vi "ReadTriggerChannelCountNode.vi"(8 "Error In":errorcluster, 11 "Trigger Node In":refnum<k20>) -> (0 "Error Out":errorcluster, 1 "Infinite?":bool, 2 "Count":u32, 3 "Trigger Node Out":refnum<k20>, 5 "Auto?":bool)   [LabVIEW 2012]
uses:
  <vilib>/xml/NI_XML.lvlib
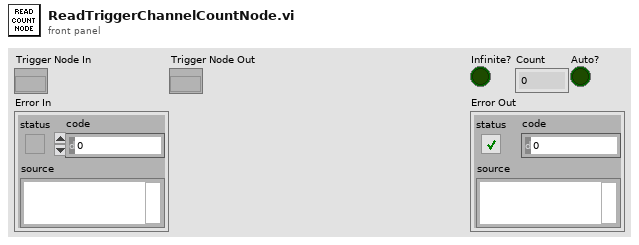
[diagram p1: front panel]
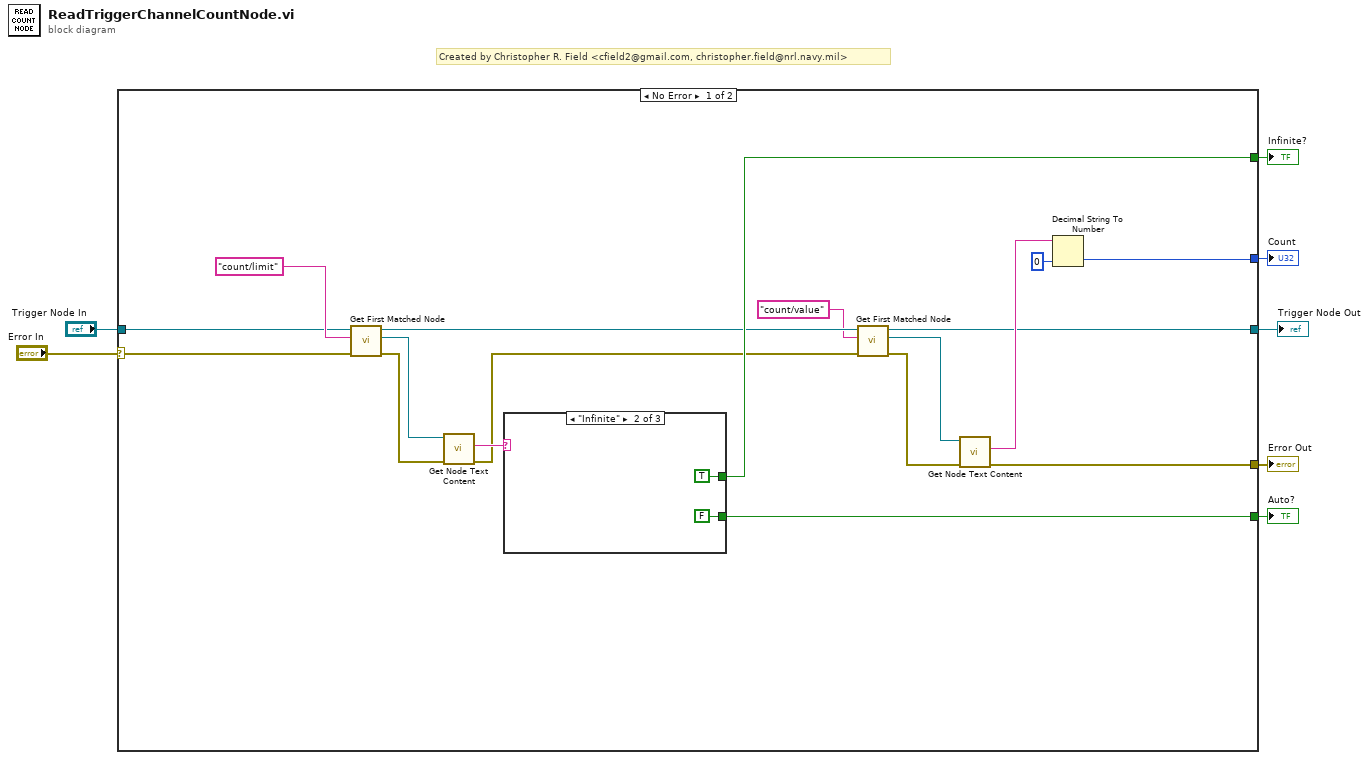
[diagram p0: block diagram]
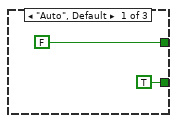
[diagram p2: hidden frame]
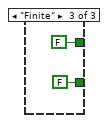
[diagram p3: hidden frame]
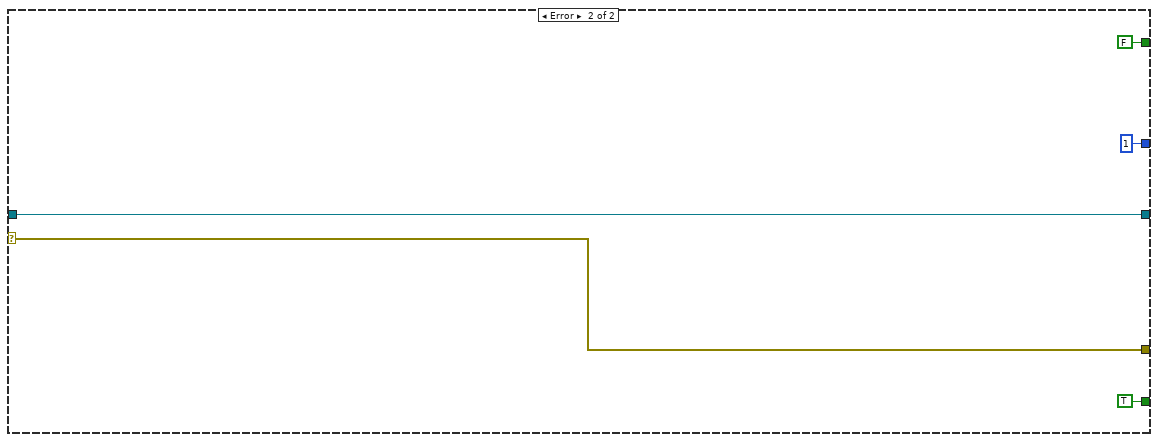
[diagram p4: hidden frame]
diagram:
  # "Created by Christopher R. Field <cfield2@gmail.com, christopher.field@nrl.navy.mil>"
  n1 = case shown="No Error" "Error In" {
    selector: "Error In" -> [w11 w36]
    tunnel: "Trigger Node In" -> [w12 w33]
    tunnel: [w21 FALSE] -> w5
    tunnel: [w13 u32 1] -> w4
    tunnel: [w10 w33] -> w3
    tunnel: [w9 w36] -> w2
    tunnel: [w8 TRUE] -> w1
    frame No Error {
      n2 = call <vilib>:"Get First Matched Node.vi"("error in (no error)"=w11, "XPath expression"="count/limit", "node in"=w12) -> ("error out"=w23:errorcluster, "node result"=w24:refnum<k20>, "node out"=w20:refnum<k20>)  [unwired: 6 in]
      n3 = call <vilib>:"Get Node Text Content.vi"("error in (no error)"=w23, "node in"=w24) -> ("error out"=w18:errorcluster, "node text"=w22:string)  [unwired: 7 in, 1 out]
      n4 = case shown="\"Infinite\"" w22 {
        tunnel: [FALSE TRUE FALSE] -> w21
        tunnel: [TRUE FALSE FALSE] -> w8
        frame "Auto", Default {
        }
        frame "Infinite" {
        }
        frame "Finite" {
        }
      }
      n5 = call <vilib>:"Get First Matched Node.vi"("error in (no error)"=w18, "XPath expression"="count/value", "node in"=w20) -> ("error out"=w16:errorcluster, "node result"=w17:refnum<k20>, "node out"=w10:refnum<k20>)  [unwired: 6 in]
      n6 = call <vilib>:"Get Node Text Content.vi"("error in (no error)"=w16, "node in"=w17) -> ("error out"=w9:errorcluster, "node text"=w15:string)  [unwired: 7 in, 1 out]
      n7 = Decimal String To Number(string=w15, default (0L)=u32 0 ("default (0 I32)")) -> (number=w13:u32)  [unwired: 1 in, 1 out]
    }
    frame Error {
    }
  }
  "Infinite?" <- w5
  "Count" <- w4
  "Trigger Node Out" <- w3
  "Error Out" <- w2
  "Auto?" <- w1
